vi "Set Configuration Directory.vi"(5 "Destination Type":string="LLB", 7 "Destination Name":string="LLB", 8 "error in (no error)":errorcluster, 10 "Directory Path":path, 11 "BuildSpec in":refnum<vi>) -> (0 "error out":errorcluster, 3 "BuildSpec out":refnum<vi>)   [LabVIEW 2019, in "Project Sync Tools.lvclass"]
uses:
  Project Sync Tools.lvclass
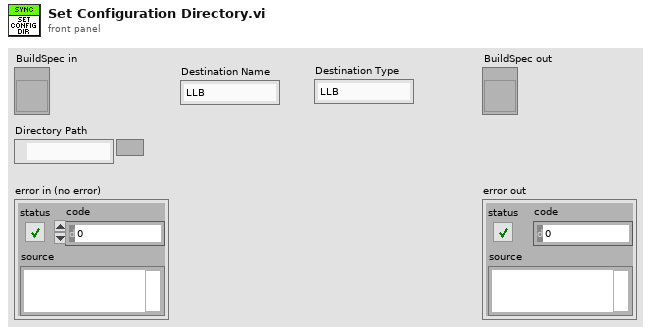
[diagram p1: front panel]
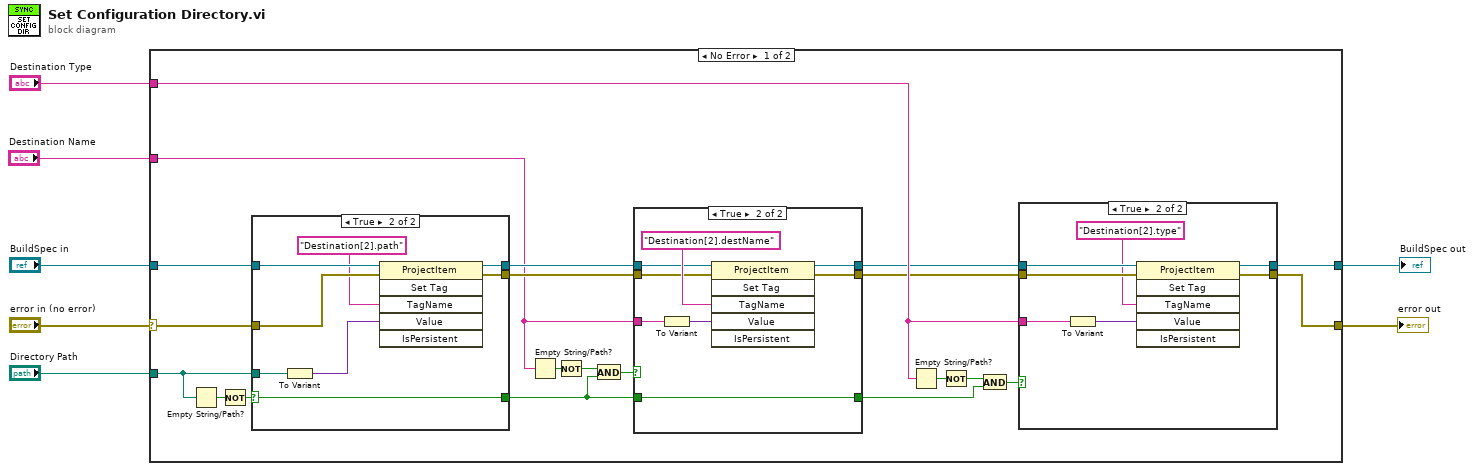
[diagram p0: block diagram]
diagram:
  n1 = case shown="No Error" "error in (no error)" {
    selector: "error in (no error)" -> [w25 w60]
    tunnel: [w28 w60] -> w7
    tunnel: [w27 w61] -> w6
    tunnel: "BuildSpec in" -> [w26 w61]
    tunnel: "Directory Path" -> [w24 _]
    tunnel: "Destination Type" -> [w23 _]
    tunnel: "Destination Name" -> [w10 _]
    frame No Error {
      n2 = Empty String/Path?(string/path=w24) -> (empty?=w22:bool)
      n3 = Not(x=w22) -> (.not. x?=w20:bool)
      n4 = case shown="True" w20 {
        selector: w20 -> [w49 w52]
        tunnel: w26 -> [w51 w59]
        tunnel: w25 -> [w50 w58]
        tunnel: w24 -> [_ w57]
        tunnel: [w50 w56] -> w15
        tunnel: [w51 w53] -> w16
        tunnel: [w49 w52] -> w9
        frame False {
        }
        frame True {
          n5 = To Variant(anything=w57) -> (Variant=w54:variant)
          n6 = invoke class="ProjectItem" method="Set Tag"(reference=w59, error in=w58, "TagName"="Destination[2].path" ("Tag Name"), "Value"=w54) -> (reference out=w53:refnum<vi>, error out=w56:errorcluster)  [unwired: 2 in, 4 out]
        }
      }
      n7 = Empty String/Path?(string/path=w10) -> (empty?=w17:bool)
      n8 = Not(x=w17) -> (.not. x?=w12:bool)
      n9 = And(x=w12, y=w9) -> (x .and. y?=w11:bool)
      n10 = case shown="True" w11 {
        tunnel: w16 -> [w30 w38]
        tunnel: w15 -> [w29 w37]
        tunnel: [w30 w36] -> w14
        tunnel: [w29 w35] -> w13
        tunnel: w10 -> [_ w34]
        tunnel: w9 -> [w31 w32]
        tunnel: [w31 w32] -> w8
        frame False {
        }
        frame True {
          n11 = To Variant(anything=w34) -> (Variant=w33:variant)
          n12 = invoke class="ProjectItem" method="Set Tag"(reference=w38, error in=w37, "TagName"="Destination[2].destName" ("Tag Name"), "Value"=w33) -> (reference out=w36:refnum<vi>, error out=w35:errorcluster)  [unwired: 2 in, 4 out]
        }
      }
      n13 = Empty String/Path?(string/path=w23) -> (empty?=w21:bool)
      n14 = Not(x=w21) -> (.not. x?=w19:bool)
      n15 = And(x=w19, y=w8) -> (x .and. y?=w18:bool)
      n16 = case shown="True" w18 {
        tunnel: [w40 w48] -> w28
        tunnel: [w41 w47] -> w27
        tunnel: w23 -> [_ w43]
        tunnel: w13 -> [w40 w46]
        tunnel: w14 -> [w41 w45]
        frame False {
        }
        frame True {
          n17 = To Variant(anything=w43) -> (Variant=w42:variant)
          n18 = invoke class="ProjectItem" method="Set Tag"(reference=w45, error in=w46, "TagName"="Destination[2].type" ("Tag Name"), "Value"=w42) -> (reference out=w47:refnum<vi>, error out=w48:errorcluster)  [unwired: 2 in, 4 out]
        }
      }
    }
    frame Error {
    }
  }
  "error out" <- w7
  "BuildSpec out" <- w6
